vi "Get Number Of Neopixels.vi"(11 "Neopixel - FPGA In":refnum<class "Neopixel - FPGA.lvclass">) -> (1 "Valid":bool, 2 "Number Of Neopixels":u16, 3 "Neopixel - FPGA Out":refnum<class "Neopixel - FPGA.lvclass">)   [LabVIEW 2021, in "Neopixel - FPGA.lvclass"]
uses:
  Neopixel - FPGA.lvclass
  Neopixel - FPGA.lvclass/Neopixel - FPGA.ctl
  <vilib>/rvi/DataTransferAndStorage/Container/Common/niFpgaContainerExecOnDevCompGetState.vi
  <vilib>/rvi/Emulation/niFpgaEmulationIsFPGAContextNoSignature.vi
  <vilib>/rvi/DataTransferAndStorage/Container/Common/niFpgaContainerGetUniqueNameForEmu.vi
  <vilib>/rvi/Memory/Memory_Emulation/niFpgaMemoryEmulationCacheClearOnFirstRun.vi
  <vilib>/rvi/Memory/Memory_Emulation/nirvimemoryEmulationManagerCache_MakeExclusive.vi
  <vilib>/rvi/Memory/Memory_Emulation/niFpgaMemoryEmulationValidateCache.vi
  <vilib>/rvi/Memory/Memory_Emulation/nirvimemoryEmulationManagerCache_InsertValue.vi
  <vilib>/Utility/error.llb/Clear Errors.vi
  <vilib>/rvi/Memory/Memory_Emulation/nirvimemoryEmulationManagerCache_ReleaseExclusive.vi
  <vilib>/rvi/Memory/Memory_Emulation/nirvimemoryEmulationManagerCache_GetValue.vi
  <vilib>/rvi/Memory/Memory_Emulation/nirvimemoryEmulationManagerCache_SetValue.vi
  <vilib>/rvi/Emulation/niFpgaProcessEmulError.vi
  <vilib>/rvi/Emulation/niFpgaSctlEmulationGetInTimedLoop.vi
  <vilib>/rvi/DataTransferAndStorage/Container/XNode/niFpgaContainer.xnode
  Controls/Number Of Neopixels.ctl
  <vilib>/rvi/DataTransferAndStorage/Register/Emulation/niFpgaRegisterEmulationRefIn.vi
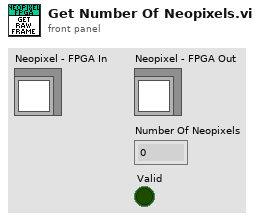
[diagram p1: front panel]
types:
  T1 = typedef "Neopixel - FPGA.lvclass/Number Of Neopixels.ctl" = refnum<k21>
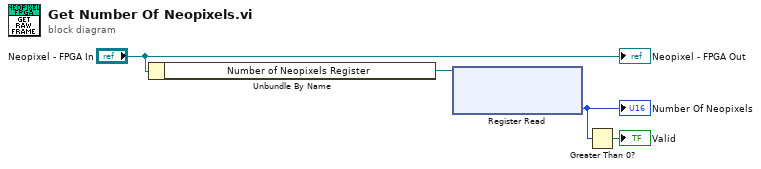
[diagram p0: block diagram]
diagram:
  n1 = Unbundle By Name("Neopixel - FPGA In") -> ("Number of Neopixels Register"=w3:T1)
  n2 = xnode ("Register Read")("Register In"=w3) -> ("Data"=w2:u16)  [unwired: 1 out]
  "Number Of Neopixels" <- w2
  n3 = Greater Than 0?(x=w2) -> (x > 0?=→"Valid":bool)
  "Neopixel - FPGA Out" <- "Neopixel - FPGA In"
